vi "DBM_WorkTime.vi"(8 "error in (no error)":errorcluster, 11 "DBManager in":refnum<class "DBManager.lvclass">) -> (0 "error out":errorcluster, 2 "date time rec":T1, 3 "DBManager out":refnum<class "DBManager.lvclass">)   [LabVIEW 2015, in "DBManager.lvclass"]
uses:
  DBManager.lvclass
  <vilib>/Utility/miscctls.llb/LVDateTimeRec.ctl
  DBManager.lvclass/DBManager.ctl
  <vilib>/drjdpowell/SQLite Library/SQL Statement/SQL Statement.lvclass/SQL Statement.ctl
  <vilib>/drjdpowell/SQLite Library/SQL Statement/Column I64.vi
  <vilib>/Utility/error.llb/Error Cluster From Error Code.vi
  <vilib>/drjdpowell/SQLite Library/SQL Statement/Error Message.vi
  <vilib>/drjdpowell/SQLite Library/SQL Statement/Column Timestamp.vi
  <vilib>/ErrorRing/Error Ring.xnode
  <vilib>/drjdpowell/SQLite Library/SQL Statement/SQL Statement.lvclass
  <vilib>/drjdpowell/SQLite Library/SQL Connection/Connection.lvclass
panel:
  # "Connector Pane"
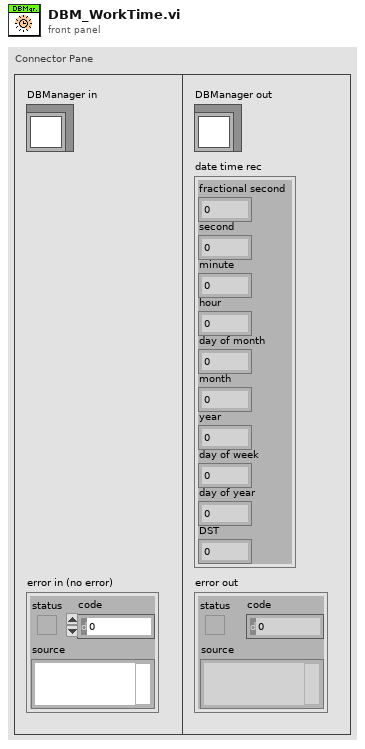
[diagram p1: front panel]
types:
  T1 = typedef "LVDateTimeRec.ctl" = cluster{"fractional second":dbl, "second":i32, "minute":i32, "hour":i32, "day of month":i32, "month":i32, "year":i32, "day of week":i32, "day of year":i32, "DST":i32}
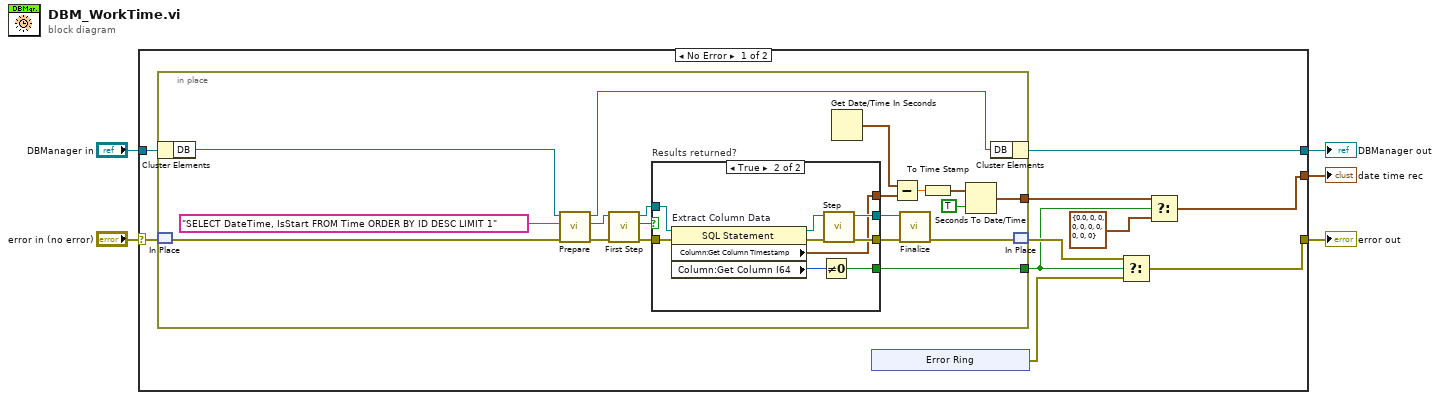
[diagram p0: block diagram]
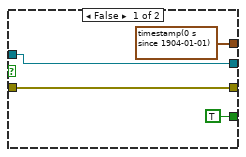
[diagram p2: hidden frame]
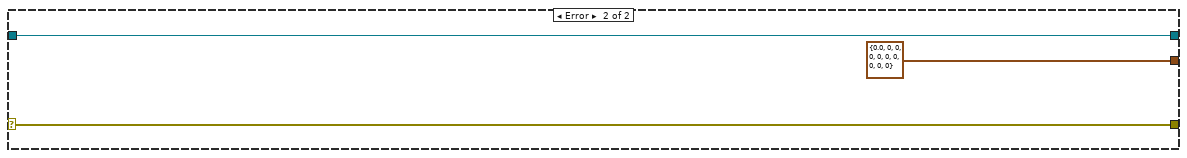
[diagram p3: hidden frame]
diagram:
  n1 = case shown="No Error" "error in (no error)" {
    selector: "error in (no error)" -> [w14 w55]
    tunnel: [w10 w55] -> w4
    tunnel: [w13 w54] -> w2
    tunnel: "DBManager in" -> [w15 w54]
    tunnel: [w6 T1 {"fractional second"=0.0, "second"=0, "minute"=0, "hour"=0, "day of month"=0, "month"=0, "year"=0, "day of week"=0, "day of year"=0, "DST"=0} ("date time rec")] -> w1
    frame No Error {
      n2 = in-place {
        in-place-border: [w22] -> w9
        in-place-border: [w27] -> w8
        n3 = in-place-cluster #1(w15) -> ("DB"=w28:refnum<class "Connection.lvclass">)
        n4 = in-place-match #2(w14) -> (w31:errorcluster)
        n5 = call <vilib>:"Prepare.vi"("error in (no error)"=w31, "SQL"="SELECT DateTime, IsStart FROM Time ORDER BY ID DESC LIMIT 1" ("SELECT  statement"), "SQLite Connection in"=w28) -> ("error out"=w35:errorcluster, "SQL Statement out"=w36:refnum<class "SQL Statement.lvclass">, "SQLite Connection out"=w29:refnum<class "Connection.lvclass">)  [unwired: 4 in, 2 out]
        n6 = call <vilib>:"First Step.vi"("error in (no error)"=w35, "SQL Statement in"=w36) -> ("error out"=w38:errorcluster, "Row returned"=w39:bool, "SQL Statement out"=w37:refnum<class "SQL Statement.lvclass">)  [unwired: 7 in]
        n7 = case "Results returned?" shown="True" w39 {
          tunnel: [w43 w52] -> w33
          tunnel: [w42 w51] -> w32
          tunnel: w37 -> [w43 w50]
          tunnel: w38 -> [w42 w49]
          tunnel: [timestamp(0 s since 1904-01-01) ("Column:Get Column Timestamp") w46] -> w25
          tunnel: [TRUE w44] -> w27
          frame False {
          }
          frame True {
            n8 = property on="Extract Column Data" class="SQL Statement"(reference=w50, error in=w49) -> (reference out=w48:refnum<class "SQL Statement.lvclass">, error out=w47:errorcluster, "Column:Get Column Timestamp"=w46:timestamp, "Column:Get Column I64"=w45:i64)
            n9 = Not Equal To 0?(x=w45) -> (x != 0?=w44:bool)
            n10 = call <vilib>:"Step.vi"("error in (no error)"=w47, "SQL Statement in"=w48) -> ("error out"=w51:errorcluster, "SQL Statement out"=w52:refnum<class "SQL Statement.lvclass">)  [unwired: 7 in, 1 out]
          }
        }
        n11 = Get Date/Time In Seconds() -> (seconds since 1Jan1904=w26:timestamp)
        n12 = Subtract(x=w26, y=w25) -> (x-y=w24:dbl)
        n13 = call <vilib>:"Finalize.vi"("error in (no error)"=w32, "SQL Statement in"=w33) -> ("error out"=w30:errorcluster)  [unwired: 9 in]
        n14 = To Time Stamp(1:w24) -> (0:w23:timestamp)
        n15 = Seconds To Date/Time(time stamp (now)=w23, to UTC (F)=TRUE) -> (date time rec=w22:T1)
        n16 = in-place-cluster #1("DB"=w29) -> (w13:refnum<class "DBManager.lvclass">)
        n17 = in-place-match #2(w30) -> (w12:errorcluster)
      }
      n18 = xnode "Error Ring"() -> ("error out"=w11:errorcluster)
      n19 = Select(t=w12, s=w8, f=w11) -> (s? t:f=w10:errorcluster)
      n20 = Select(t=w9, s=w8, f=T1 {"fractional second"=0.0, "second"=0, "minute"=0, "hour"=0, "day of month"=0, "month"=0, "year"=0, "day of week"=0, "day of year"=0, "DST"=0}) -> (s? t:f=w6:T1)
    }
    frame Error {
    }
  }
  "error out" <- w4
  "DBManager out" <- w2
  "date time rec" <- w1
